vi "Initiate Measurement Continuous.vi"(8 "error in (no error)":errorcluster, 10 "Enable Continuous (T: Enable)":bool=TRUE, 11 "VISA resource name":refnum<visa-resource-name>) -> (0 "error out":errorcluster, 3 "VISA resource name out":refnum<visa-resource-name>)   [LabVIEW 2013, in "DmmPwr Simulator.lvlib"]
doc: "Specifies whether you want to enable the initiate continuous measurement.\n\n<B>Note:</B>\n\nThis VI does not check the instrument status. Typically, you call this VI only in a sequence of calls to other low-level instrument driver VIs. The sequence performs one operation. You use the low-level VIs to optimize one or more aspects of interaction with the instrument. If you want to check the instrument status, call the <B>Error Query VI</B> at the conclusion of the sequence."
uses:
  <instrlib>/DmmPwr Simulator/DmmPwr Simulator.lvlib
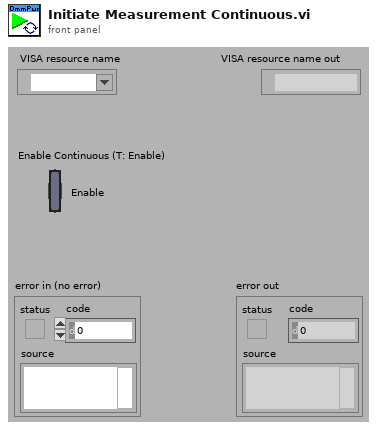
[diagram p1: front panel]
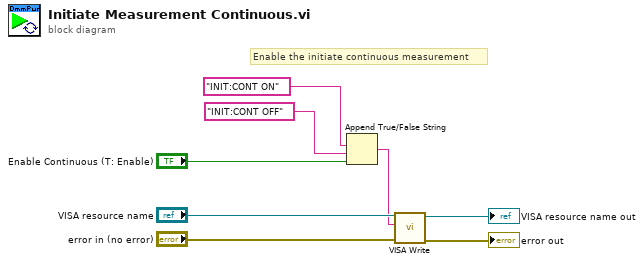
[diagram p0: block diagram]
diagram:
  # "Enable the initiate continuous measurement"
  n1 = Append True/False String(1:"Enable Continuous (T: Enable)", 2:"INIT:CONT OFF", 3:"INIT:CONT ON") -> (0:w1:string)  [unwired: 1 out]
  n2 = call <instrlib>:"VISA Write.vi"("error in"="error in (no error)", "write buffer"=w1, "VISA resource name"="VISA resource name") -> ("error out"=→"error out":errorcluster, "VISA resource name out"=→"VISA resource name out":refnum<visa-resource-name>)  [unwired: 6 in, 1 out]
